vi "M14_Control_Panel_Globals.vi"() -> ()   [LabVIEW 2019]
panel:
  in  "Control_Panel":string="Control_Panel"
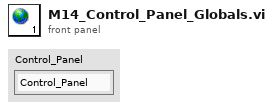
[diagram p1: front panel]
diagram:
